vi "getSerializedData.vi"(0 "reference":refnum<class "SegmentedLineEdge.lvclass">, 5 "error in (no error)":errorcluster) -> (14 "reference out":refnum<class "SegmentedLineEdge.lvclass">, 15 "startNode":refnum<class "AbstractNode.lvclass">, 16 "endNode":refnum<class "AbstractNode.lvclass">, 17 "xmlOut":string, 19 "error out":errorcluster)   [LabVIEW 2012, in "SegmentedLineEdge.lvclass"]
doc: "getSerializedData"
uses:
  <resource>/Framework/Providers/Open_GDS/UML/SegmentedLineEdge_class/SegmentedLineEdge.lvclass
  <resource>/Framework/Providers/Open_GDS/UML/AbstractNode_class/AbstractNode.lvclass
  <resource>/Framework/Providers/Open_GDS/UML/AbstractNode_class/ObjectReference.ctl
  <resource>/Framework/Providers/Open_GDS/UML/LineStyle_class/ObjectReference.ctl
  <resource>/Framework/Providers/Open_GDS/UML/ArrowHead_class/ObjectReference.ctl
  <resource>/Framework/Providers/Open_GDS/UML/General/Point/Point Point2D.ctl
  <resource>/Framework/Providers/Open_GDS/UML/ArrowHead_class/ArrowHead.lvclass
  <resource>/Framework/Providers/Open_GDS/UML/LineStyle_class/LineStyle.lvclass
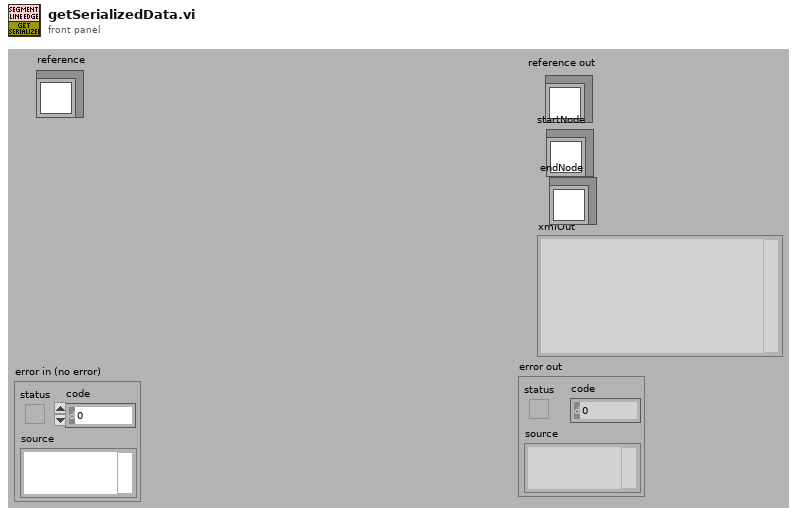
[diagram p1: front panel]
types:
  T1 = typedef "AbstractNode.lvclass/ObjectReference.ctl" = refnum<k1>
  T2 = typedef "LineStyle.lvclass/ObjectReference.ctl" = refnum<k1>
  T3 = typedef "ArrowHead.lvclass/ObjectReference.ctl" = refnum<k1>
  T4 = typedef "Point Point2D.ctl" = cluster{"x":dbl, "y":dbl}
  T5 = cluster{"Base class":cluster{"Base class":cluster{"start":T1, "end":T1}}, "lineStyle":T2, "startArrowHead":T3, "endArrowHead":T3, "startLabel":string, "midLabel":string, "endLabel":string, "MidLabelOffset":T4, "SplitWire":bool}
  T6 = typedef "SegmentedLineEdge.lvclass/ObjectAttributes.ctl" = cluster{"Base class":T7, "lineStyle":refnum<class "LineStyle.lvclass">, "startArrowHead":refnum<class "ArrowHead.lvclass">, "endArrowHead":refnum<class "ArrowHead.lvclass">, "startLabel":string, "midLabel":string, "endLabel":string, "MidLabelOffset":T4, "SplitWire":bool}
  T7 = typedef "GeneralPathEdge.lvclass/ObjectAttributes.ctl" = cluster{"Base class":T8}
  T8 = typedef "AbstractEdge.lvclass/ObjectAttributes.ctl" = cluster{"start":refnum<class "AbstractNode.lvclass">, "end":refnum<class "AbstractNode.lvclass">}
  T9 = cluster{"Base class":cluster{"Base class":cluster{"Base class":cluster{"start":T1, "end":T1}}, "lineStyle":T2, "startArrowHead":T3, "endArrowHead":T3, "startLabel":string, "midLabel":string, "endLabel":string, "MidLabelOffset":T4, "SplitWire":bool}, "Type(String)":string, "Object name":string, "Object name":string}
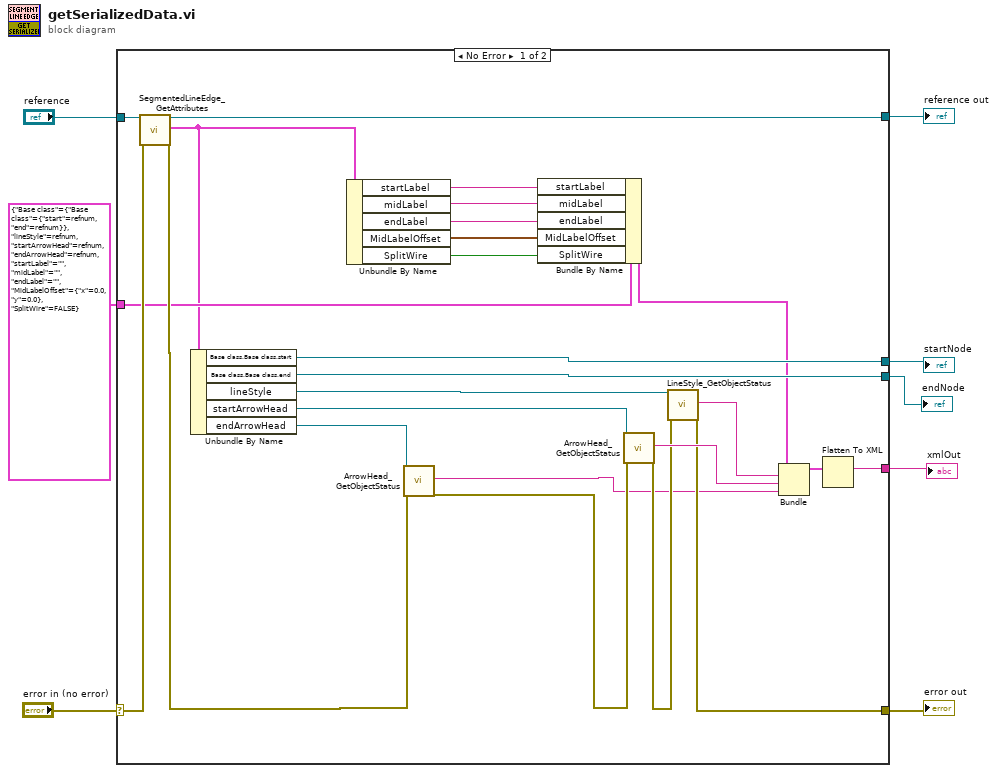
[diagram p0: block diagram]
diagram:
  n1 = case shown="No Error" "error in (no error)" {
    selector: "error in (no error)" -> [w33 w34]
    tunnel: "reference" -> [w32 w35]
    tunnel: [w19 w34] -> w6
    tunnel: [w31 w35] -> w5
    tunnel: [w29 _] -> w4
    tunnel: [w28 _] -> w3
    tunnel: [w27 _] -> w2
    tunnel: T5 {"Base class"={"Base class"={"start"=refnum, "end"=refnum}}, "lineStyle"=refnum, "startArrowHead"=refnum, "endArrowHead"=refnum, "startLabel"="", "midLabel"="", "endLabel"="", "MidLabelOffset"={"x"=0.0, "y"=0.0}, "SplitWire"=FALSE} ("Base class") -> [w11 _]
    frame No Error {
      n2 = call <resource>:"SegmentedLineEdge_GetAttributes.vi"("reference in"=w32, "error in (no error)"=w33) -> ("reference out"=w31:refnum<class "SegmentedLineEdge.lvclass">, "Attributes"=w10:T6, "error out"=w17:errorcluster)  [unwired: 15 out]
      n3 = Unbundle By Name(w10) -> ("Base class.Base class.start"=w28:refnum<class "AbstractNode.lvclass">, "Base class.Base class.end"=w27:refnum<class "AbstractNode.lvclass">, "lineStyle"=w26:refnum<class "LineStyle.lvclass">, "startArrowHead"=w24:refnum<class "ArrowHead.lvclass">, "endArrowHead"=w23:refnum<class "ArrowHead.lvclass">)
      n4 = Unbundle By Name(w10) -> ("startLabel"=w16:string, "midLabel"=w15:string, "endLabel"=w14:string, "MidLabelOffset"=w13:T4, "SplitWire"=w12:bool)
      n5 = call <resource>:"ArrowHead_GetObjectStatus.vi"("reference in"=w23, "error in (no error)"=w17) -> ("Object name"=w18:string, "error out"=w21:errorcluster)  [unwired: 16 out]
      n6 = Bundle By Name(cluster=w11, "startLabel"=w16, "midLabel"=w15, "endLabel"=w14, "MidLabelOffset"=w13, "SplitWire"=w12) -> (w9:T5)
      n7 = call <resource>:"ArrowHead_GetObjectStatus.vi"("reference in"=w24, "error in (no error)"=w21) -> ("Object name"=w22:string, "error out"=w20:errorcluster)  [unwired: 16 out]
      n8 = call <resource>:"LineStyle_GetObjectStatus.vi"("reference"=w26, "error in (no error)"=w20) -> ("Type(String)"=w25:string, "error out"=w19:errorcluster)  [unwired: 15 in, 1 out]
      n9 = Bundle("Base class"=w9, "Type(String)"=w25, "Object name"=w22, "Object name"=w18) -> (w30:T9)  [unwired: 1 out]
      n10 = Flatten To XML(anything=w30) -> (xml string=w29:string)
    }
    frame Error {
    }
  }
  "reference out" <- w5
  "error out" <- w6
  "startNode" <- w3
  "endNode" <- w2
  "xmlOut" <- w4
